vi "NotifyOwner(Message).vi"(8 "error in (no error)":errorcluster, 9 "Payload":variant, 10 "Message (empty : payload label)":string, 11 "SMO in":refnum<class "SMO.lvclass">) -> (0 "error out":errorcluster, 3 "SMO out":refnum<class "SMO.lvclass">)   [LabVIEW 2013, in "SMO.lvclass"]
uses:
  SMO.lvclass
  Support/Attribute.Owner/Attribute.Owner.lvclass
  Support/Attribute/Attribute.lvclass
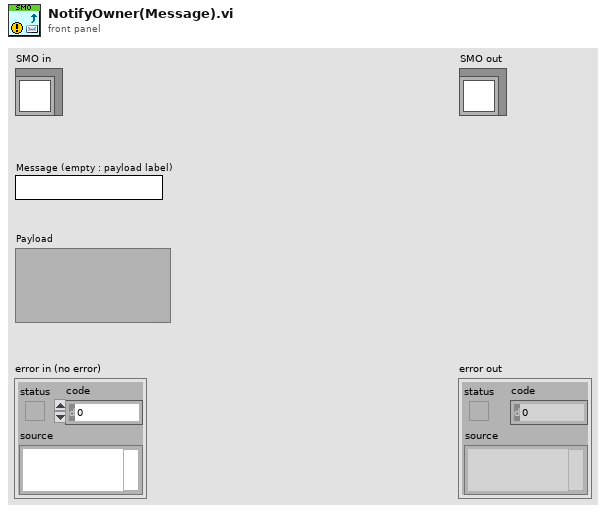
[diagram p1: front panel]
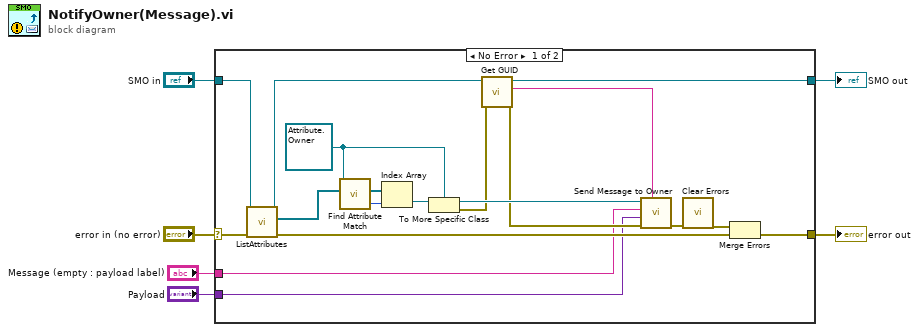
[diagram p0: block diagram]
diagram:
  n1 = case shown="No Error" "error in (no error)" {
    selector: "error in (no error)" -> [w23 w27]
    tunnel: [w15 w27] -> w5
    tunnel: [w13 w26] -> w3
    tunnel: "SMO in" -> [w24 w26]
    tunnel: "Message (empty : payload label)" -> [w8 _]
    tunnel: "Payload" -> [w7 _]
    frame No Error {
      w14 = refnum<class "Attribute.Owner.lvclass"> refnum ("Attribute.Owner.lvclass")
      n2 = call "ListAttributes.vi"("error in (no error)"=w23, "SMO in"=w24) -> ("error out"=w16:errorcluster, "[Attributes]"=w25:refnum<class "Attribute.lvclass">[], "SMO out"=w11:refnum<class "SMO.lvclass">)  [unwired: 7 in]
      n3 = call "Find Attribute Match.vi"("Attributes"=w25, "Attribute in"=w14) -> ("Matched index"=w21:i32, "Attributes dup"=w22:refnum<class "Attribute.lvclass">[])  [unwired: 7 in, 1 out]
      n4 = Index Array(array=w22, index=w21) -> (element=w20:refnum<class "Attribute.lvclass">)
      n5 = To More Specific Class(target class=w14, reference=w20) -> (specific class reference=w19:refnum<class "Attribute.Owner.lvclass">, error out=w10:errorcluster)  [unwired: 1 in]
      n6 = call "Get GUID.vi"("error in (no error)"=w10, "SMO"=w11) -> ("error out"=w12:errorcluster, "GUID"=w9:string, "SMO out"=w13:refnum<class "SMO.lvclass">)  [unwired: 7 in]
      n7 = call "Send Message to Owner.vi"("GUID"=w9, "error in (no error)"=w12, "Message Payload"=w7, "Message"=w8, "Attribute.Owner in"=w19) -> ("error out"=w18:errorcluster)  [unwired: 5 in, 1 out]
      n8 = call <vilib>:"Clear Errors.vi"("error in (no error)"=w18) -> ("error out"=w17:errorcluster)  [unwired: 6 in]
      n9 = Merge Errors(w17, w16) -> (w15:errorcluster)
    }
    frame Error {
    }
  }
  "error out" <- w5
  "SMO out" <- w3
